vi "example_01_load_from_xml.vi"() -> ()   [LabVIEW 2015, in "lv-unit-conversion.lvlib"]
uses:
  lv-unit-conversion.lvlib
  public/_controls/unit_set.ctl
panel:
  out "unit_set":variant
  out "units []":T1[](array[typedef])
  out "raw_data []":T2(array[cluster])
  in  "symbols []":string[](array[string])
  out "error out":errorcluster
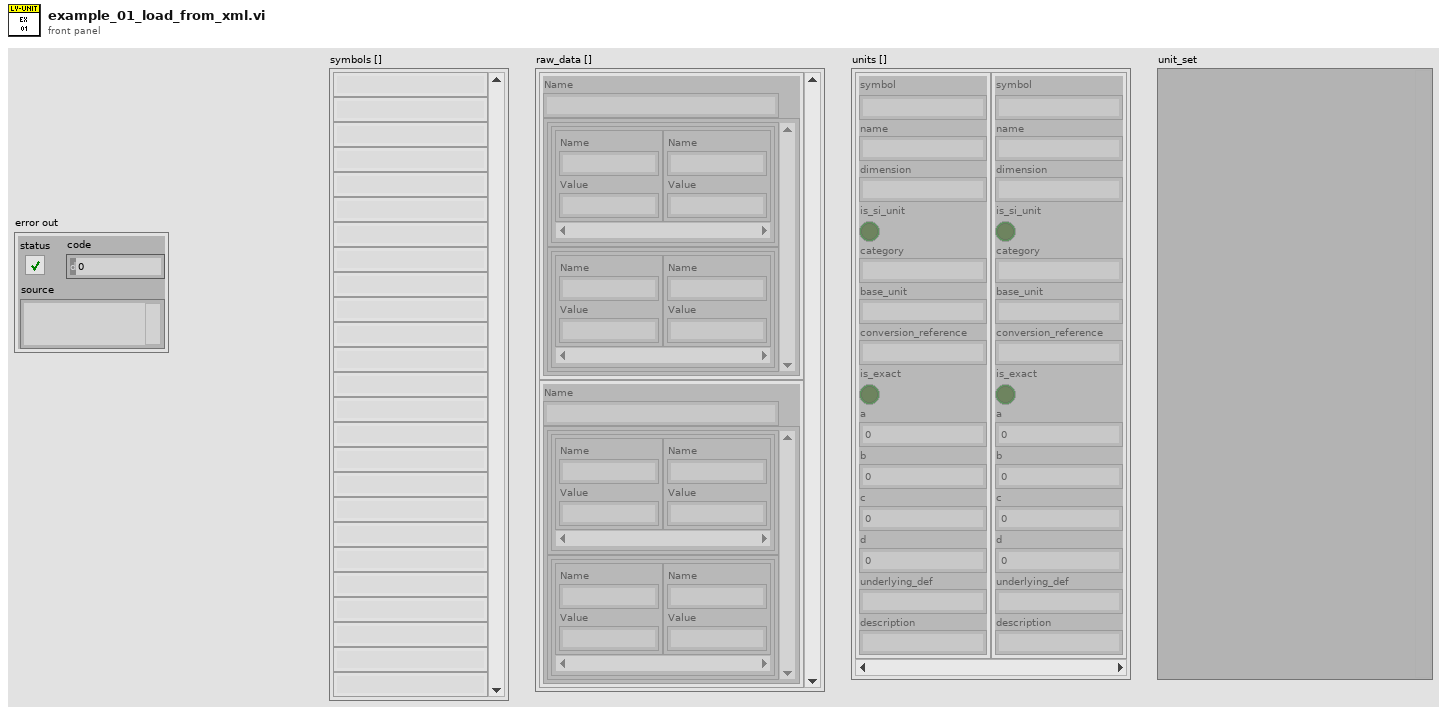
[diagram p1: front panel]
types:
  T1 = typedef "lv-unit-conversion.lvlib/unit_set.ctl" = cluster{"symbol":string, "name":string, "dimension":string, "is_si_unit":bool, "category":string, "base_unit":string, "conversion_reference":string, "is_exact":bool, "a":dbl, "b":dbl, "c":dbl, "d":dbl, "underlying_def":string, "description":string}
  T2 = cluster{"Name":string, cluster{cluster{"Name":string, "Value":string}[]}[]}[]
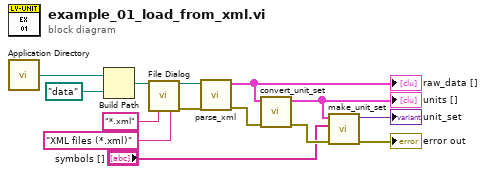
[diagram p0: block diagram]
diagram:
  n1 = call <vilib>:"Application Directory.vi"() -> ("Application Directory"=w10:path)
  n2 = Build Path(base path=w10, name or relative path=path "data" ("Application Directory")) -> (appended path=w8:path)
  n3 = call "File Dialog"("start path"=w8, "pattern (all files)"="*.xml", "pattern label"="XML files (*.xml)") -> ("selected path"=w5:path, "error out"=w4:errorcluster)  [unwired: 9 in, 2 out]
  n4 = call "parse_xml.vi"("error in (no error)"=w4, "XML File Path"=w5) -> ("error out"=w13:errorcluster, "raw_data []"=w14:cluster{"Name":string, cluster{cluster[]}[]}[])  [unwired: 8 in]
  "raw_data []" <- w14
  n5 = call "convert_unit_set.vi"("error in (no error)"=w13, "raw_data []"=w14) -> ("error out"=w11:errorcluster, "units []"=w12:T1[])  [unwired: 8 in]
  "units []" <- w12
  n6 = call "make_unit_set.vi"("error in (no error)"=w11, "symbols []"="symbols []", "units []"=w12) -> ("error out"=→"error out":errorcluster, "unit_set out"=→"unit_set":variant)  [unwired: 7 in]
